vi "LickSpoutPrimer.vi"() -> ()   [LabVIEW 2019]
doc: "The myRIO Project template acquires acceleration data from the onboard accelerometer and displays the changes of acceleration values in a waveform chart."
uses:
  <vilib>/myRIO/Common/Instrument Driver Framework/myRIO v1.0/Encoder/typedefs/Encoder Signal Mode.ctl
  <vilib>/myRIO/Instrument Drivers/Onboard IO/Encoder/typedefs/Encoder Reference.ctl
  <vilib>/myRIO/Common/Instrument Driver Framework/Utilities/typedefs/myRIO Generic Hardware Reference.ctl
  <vilib>/myRIO/Common/Instrument Driver Framework/Utilities/typedefs/Hardware Version Enum.ctl
  <vilib>/myRIO/Common/Instrument Driver Framework/Utilities/typedefs/myRIO v1.0 Reference.ctl
  <vilib>/myRIO/Common/Instrument Driver Framework/Utilities/typedefs/Generic FPGA Reference.ctl
  <vilib>/myRIO/Common/Instrument Driver Framework/myRIO v1.0/Encoder/typedefs/Encoder Channels Enum.ctl
  <vilib>/myRIO/Common/Instrument Driver Framework/myRIO v1.0/Encoder/typedefs/Encoder Configuration v1.0.ctl
  <vilib>/userdefined/High Color/nirio_resource_hc.ctl
  <vilib>/myRIO/Instrument Drivers/Onboard IO/DIO/typedefs/DIO Reference.ctl
  <vilib>/myRIO/Common/Instrument Driver Framework/myRIO v1.0/DIO/typedefs/DIO Channels List.ctl
  <vilib>/myRIO/Common/Instrument Driver Framework/myRIO v1.0/DIO/typedefs/DIO Channels Enum.ctl
  <vilib>/myRIO/Common/Instrument Driver Framework/Utilities/vis/Is FPGA Ref Available.vi
  <vilib>/myRIO/Common/Instrument Driver Framework/myRIO v1.0/Encoder/vis/myRIO v1.1 Open Encoder.vi
  <vilib>/myRIO/Instrument Drivers/Onboard IO/Encoder/vis/Read.vi
  <vilib>/myRIO/Common/Instrument Driver Framework/myRIO v1.0/DIO/vis/myRIO v1.1 Open DIO.vi
  <vilib>/myRIO/Instrument Drivers/Onboard IO/DIO/vis/Read.vi
  <vilib>/myRIO/Instrument Drivers/Onboard IO/DIO/vis/Write.vi
  <vilib>/myRIO/Common/Instrument Driver Framework/Utilities/vis/Validate Channels.vi
  <vilib>/myRIO/Common/Instrument Driver Framework/myRIO v1.0/Encoder/vis/myRIO v1.0 Reserve Encoder.vi
  <vilib>/myRIO/Common/Instrument Driver Framework/myRIO v1.0/DIO/vis/myRIO v1.0 Reserve DIO.vi
  <vilib>/myRIO/Common/Instrument Driver Framework/myRIO v1.0/Encoder/vis/myRIO v1.0 Build MUX Configuration Encoder.vi
  <vilib>/myRIO/Common/Instrument Driver Framework/myRIO v1.0/Resource Manager/vis/myRIO v1.0 Reserve Channel List.vi
  <vilib>/myRIO/Common/Instrument Driver Framework/myRIO v1.0/DIO/vis/myRIO v1.0 Build MUX Configuration DIO.vi
  <vilib>/myRIO/Common/Instrument Driver Framework/myRIO v1.0/Resource Manager/vis/myRIO v1.0 Create Configuration List.vi
  <vilib>/myRIO/Common/Instrument Driver Framework/myRIO v1.0/Resource Manager/vis/myRIO v1.0 Reserve Channel.vi
  <vilib>/myRIO/Common/Instrument Driver Framework/myRIO v1.0/Resource Manager/vis/myRIO v1.0 Unreserve Channel.vi
  <vilib>/myRIO/Common/Instrument Driver Framework/myRIO v1.0/Resource Manager/vis/myRIO v1.0 Build Mutex Name.vi
  <vilib>/Utility/VariantDataType/GetNumericInfo.vi
  <vilib>/Utility/error.llb/Error Cluster From Error Code.vi
  <vilib>/myRIO/Common/Instrument Driver Framework/myRIO v1.0/myRIO v1.1 Open.vi
  <vilib>/myRIO/Common/Instrument Driver Framework/Utilities/vis/IO Manager.vi
  <vilib>/myRIO/Common/Instrument Driver Framework/Utilities/vis/Configuration Manager.vi
  <vilib>/myRIO/Common/Instrument Driver Framework/myRIO v1.0/Resource Manager/vis/myRIO v1.0 Configure IO.vi
  <vilib>/myRIO/Common/Instrument Driver Framework/myRIO v1.0/myRIO v1.0 Close.vi
  <vilib>/myRIO/Common/Instrument Driver Framework/myRIO v1.0/Encoder/vis/myRIO v1.0 Configure Encoder.vi
  <vilib>/myRIO/Common/Instrument Driver Framework/myRIO v1.0/Encoder/vis/myRIO v1.0 Read Encoder.vi
  <vilib>/myRIO/Common/Instrument Driver Framework/myRIO v1.0/DIO/vis/myRIO v1.0 Read DIO.vi
  <vilib>/myRIO/Common/Instrument Driver Framework/myRIO v1.0/DIO/vis/myRIO v1.0 Write DIO.vi
  <vilib>/myRIO/Express VI/Onboard IO/Encoder/Encoder Express VI.xnode
  <vilib>/myRIO/Instrument Drivers/Onboard IO/Encoder/vis/myRIO Encoder Open.xnode
  <vilib>/myRIO/Express VI/Onboard IO/DI/DI Express VI.xnode
  <vilib>/myRIO/Instrument Drivers/Onboard IO/DIO/vis/myRIO DIO Open.xnode
  <vilib>/myRIO/Express VI/Onboard IO/DO/DO Express VI.xnode
  <vilib>/myRIO/Instrument Drivers/Onboard IO/Encoder/Encoder.lvlib
  <vilib>/myRIO/Instrument Drivers/Onboard IO/DIO/DIO.lvlib
panel:
  in  "Stop Button":bool
  out "Time since last reward":dbl
  out "Time of last reward":dbl
  out "Rewards":u16
  out "Frame clock":i32
  out "Frames":u32
  out "Reward":bool=TRUE
  in  "Give reward":bool
  out "Licks":u32
  out "Lick":bool
  out "Output":dbl[][](array[numeric])
  out "Time":dbl
  out "Display":bool
  out "Overflow?":bool
  out "Counter Value":i32
  out "Velocity":dbl
  out "Velocity Plot":dbl[](graph)
  out "Velocity array":dbl[](array[numeric])
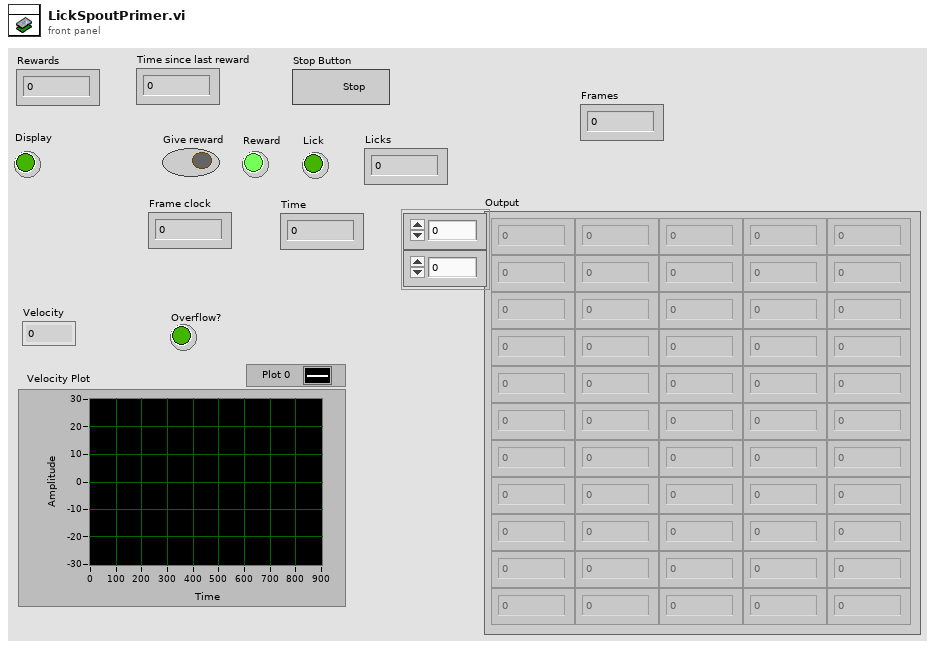
[diagram p1: front panel]
types:
  T1 = typedef "Encoder.lvlib/Encoder Reference.ctl" = cluster{"myRIO Reference":T2, "Encoder Channels Enum":T6}
  T2 = typedef "myRIO Generic Hardware Reference.ctl" = cluster{"myRIO Model":T3, "myRIO Hardware Reference":T4}
  T3 = typedef "Hardware Version Enum.ctl" = enum16{"Unknown", "myRIO-1900", "myRIO-1950", "roboRIO", "NI ELVIS RIO CM", "ELVIS III"}
  T4 = typedef "myRIO v1.0 Reference.ctl" = cluster{"Generic FPGA Reference":T5, "Allow multiple opens":bool}
  T5 = typedef "Generic FPGA Reference.ctl" = refnum<k20>
  T6 = typedef "Encoder Channels Enum.ctl" = enum16{"Not Connected", "C/ENC0", "C/ENC1", "A/ENC", "A/ENC0", "A/ENC1", "A/ENC2", "A/ENC3", "A/ENC4", "A/ENC5", "A/ENC6", "A/ENC7", "A/ENC8", "A/ENC9", "B/ENC", "B/ENC0", "B/ENC1", "B/ENC2", "B/ENC3", "B/ENC4", "B/ENC5", "B/ENC6", "B/ENC7", "B/ENC8", "B/ENC9", "DIO/ENC0", "DIO/ENC1", "DIO/ENC2", "DIO/ENC3", "DIO/ENC4"}
  T7 = typedef "Encoder Signal Mode.ctl" = enum16{"Quadrature phase signal", "Step and direction signal"}
  T8 = typedef "nirio_resource_hc.ctl" = tag
  T9 = typedef "DIO.lvlib/DIO Reference.ctl" = cluster{"myRIO Reference":T2, "DIO Channels List":T10}
  T10 = typedef "DIO Channels List.ctl" = T11[]
  T11 = typedef "DIO Channels Enum.ctl" = enum16{"Not Connected", "C/DIO0", "C/DIO1", "C/DIO2", "C/DIO3", "C/DIO4", "C/DIO5", "C/DIO6", "C/DIO7", "A/DIO0", "A/DIO1", "A/DIO2", "A/DIO3", "A/DIO4", "A/DIO5", "A/DIO6", "A/DIO7", "A/DIO8", "A/DIO9", "A/DIO10", "A/DIO11", "A/DIO12", "A/DIO13", "A/DIO14", "A/DIO15", "A/DIO16", "A/DIO17", "A/DIO18", "A/DIO19", "B/DIO0", "B/DIO1", "B/DIO2", "B/DIO3", "B/DIO4", "B/DIO5", "B/DIO6", "B/DIO7", "B/DIO8", "B/DIO9", "B/DIO10", "B/DIO11", "B/DIO12", "B/DIO13", "B/DIO14", "B/DIO15", "B/DIO16", "B/DIO17", "B/DIO18", "B/DIO19", "LED0", "LED1", "LED2", "LED3", "Button0", "DIO/DIO0", "DIO/DIO1", "DIO/DIO2", "DIO/DIO3", "DIO/DIO4", "DIO/DIO5", "DIO/DIO6", "DIO/DIO7", "DIO/DIO8", "DIO/DIO9", "SPI/CS0", "SPI/CS1", "SPI/CS2", "SPI/CS3", "LED RADIO (Green)", "LED RADIO (Red)", "LED COMM (Green)", "LED COMM (Red)", "LED MODE (Green)", "LED MODE (Red)"}
  T12 = typedef "NI_Matrix.lvlib/RealMatrix.ctl" = dbl[][]
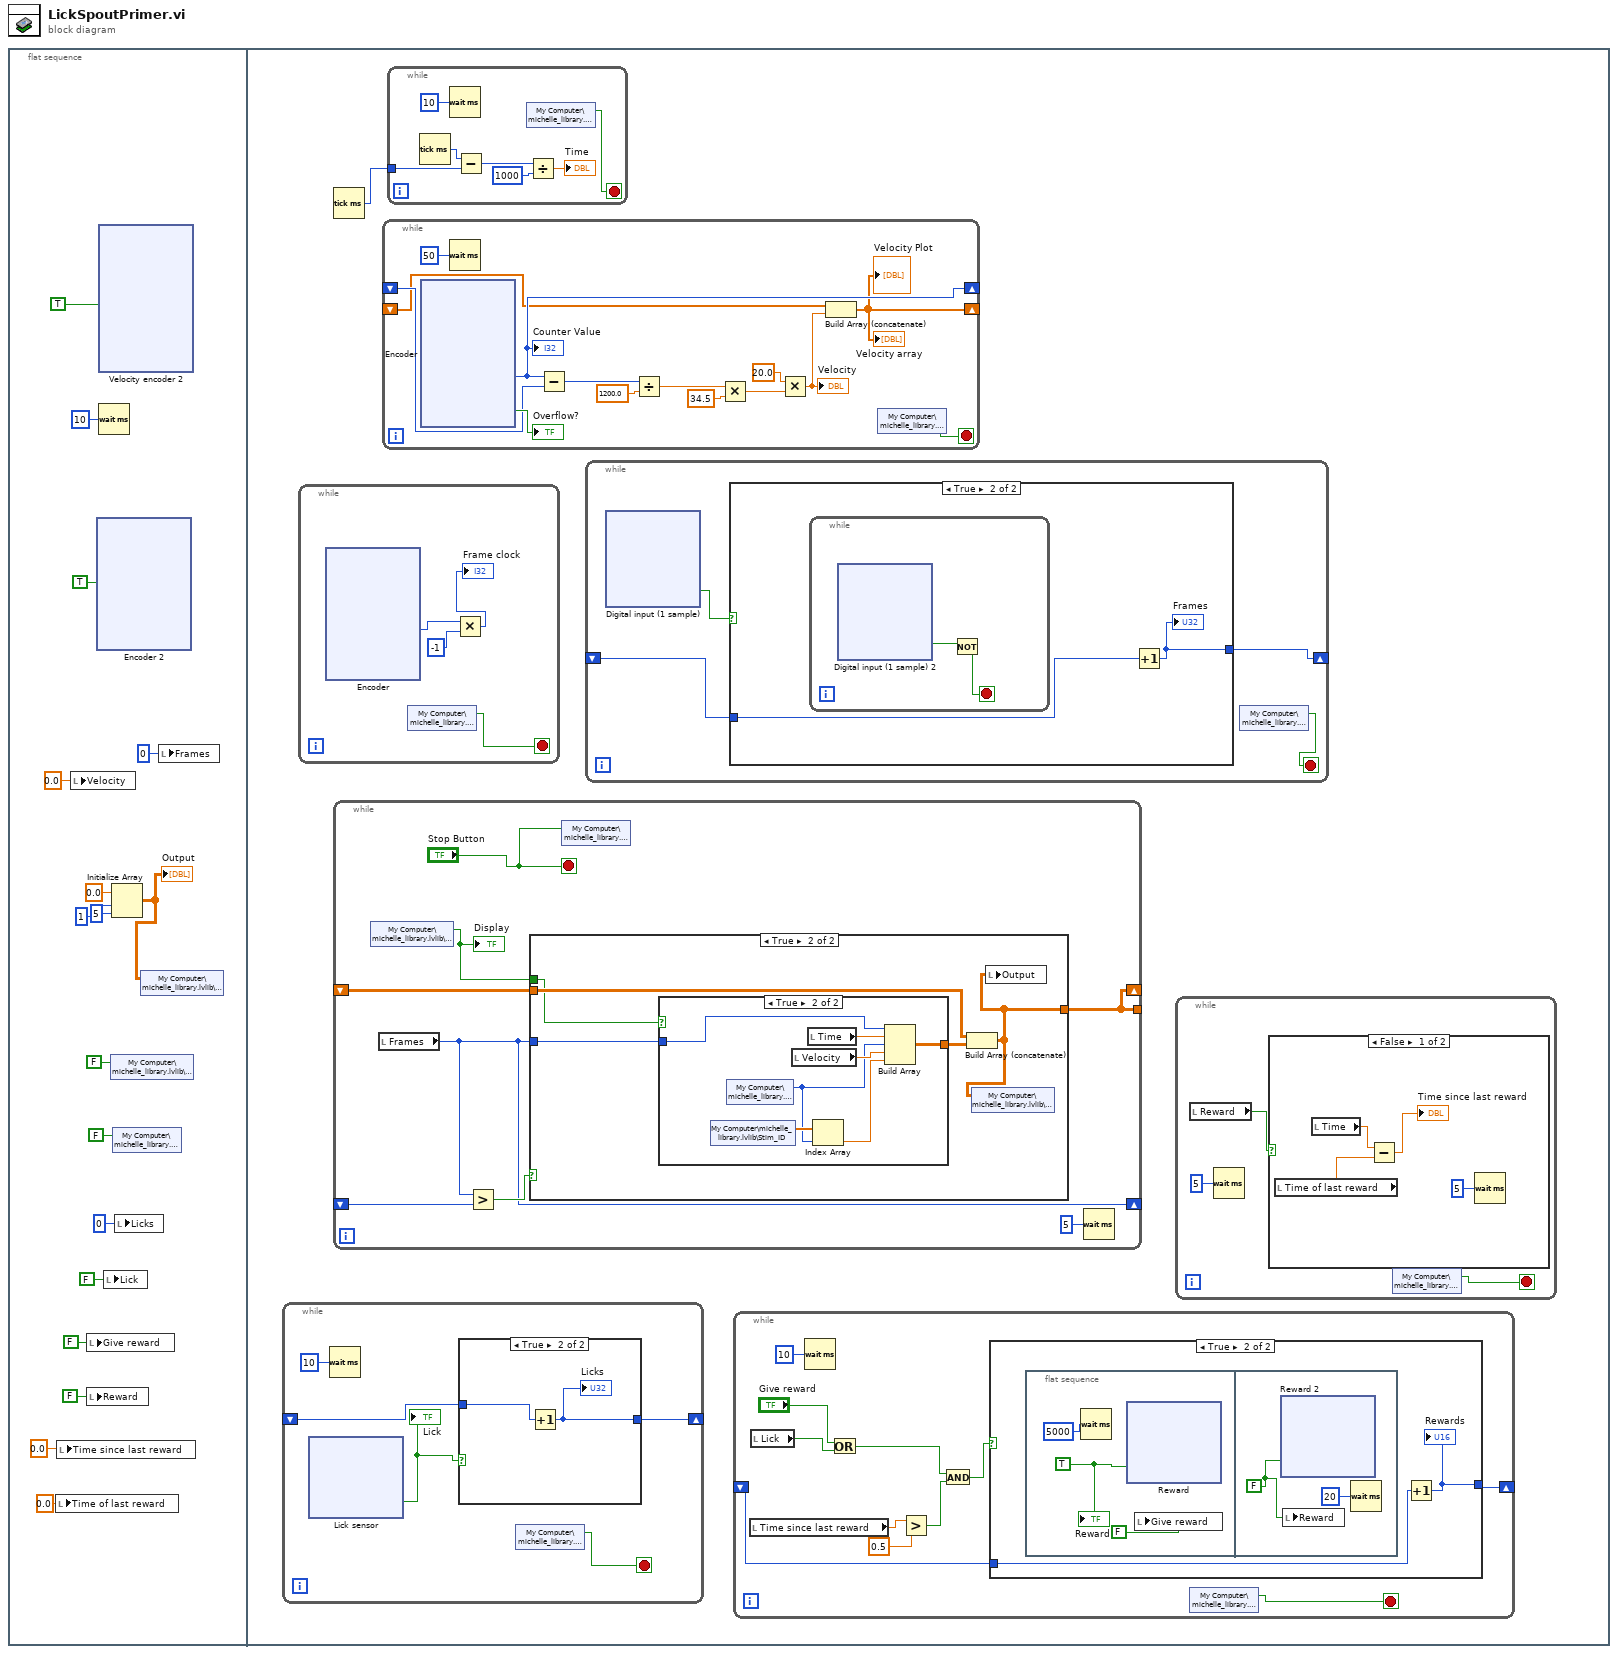
[diagram p0: block diagram]
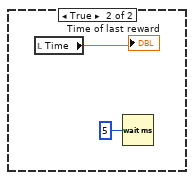
[diagram p2: hidden frame]
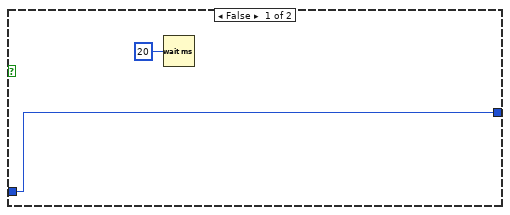
[diagram p4: hidden frame]
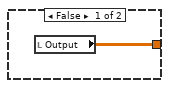
[diagram p6: hidden frame]
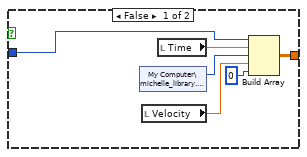
[diagram p7: hidden frame]
diagram:
  n1 = flat-sequence {
    frame #0 {
      n2 = local write "Time of last reward"(0.0 ("Time of last reward")) -> ()
      n3 = local write "Time since last reward"(0.0 ("Time since last reward")) -> ()
      n4 = local write "Velocity"(0.0 ("Velocity")) -> ()
      n5 = local write "Give reward"(FALSE ("Give reward")) -> ()
      n6 = local write "Reward"(FALSE ("Reward")) -> ()
      n7 = xnode "Encoder 2"("Reset Counter"=TRUE) -> ()  [unwired: 1 in, 4 out]
      n8 = xnode "Velocity encoder 2"("Reset Counter"=TRUE) -> ()  [unwired: 1 in, 4 out]
      n9 = Wait (ms)(milliseconds to wait=u32 10) -> ()  [unwired: 1 out]
      n10 = local write "Lick"(FALSE ("Lick")) -> ()
      n11 = shared-variable "My Computer\\michelle_library.lvlib\\Display"(FALSE ("Display")) -> ()  [unwired: 1 in, 1 out]
      n12 = Initialize Array(0.0 ("element"), 1 ("dimension size"), 5 ("dimension size")) -> (w11:dbl[][])
      "Output" <- w11
      n13 = shared-variable "My Computer\\michelle_library.lvlib\\Stop"(FALSE ("Stop")) -> ()  [unwired: 1 in, 1 out]
      n14 = local write "Licks"(u32 0 ("Licks")) -> ()
      n15 = shared-variable "My Computer\\michelle_library.lvlib\\Output"(w11) -> ()  [unwired: 1 in, 1 out]
      n16 = local write "Frames"(u32 0 ("Frames")) -> ()
    }
    frame #1 {
      n17 = while {
        shift-right: [w340] -> _
        shift-left: _ -> [w339]
        stop <- w343 stop-if-true
        n18 = xnode "Lick sensor"() -> ("C/DIO1 (DIO1)"=w341:bool)  [unwired: 1 in, 1 out]
        "Lick" <- w341
        n19 = Wait (ms)(milliseconds to wait=u32 10) -> ()  [unwired: 1 out]
        n20 = case shown="True" w341 {
          tunnel: [w344 w346] -> w340
          tunnel: w339 -> [w344 w345]
          frame False {
          }
          frame True {
            n21 = Increment(x=w345) -> (x+1=w346:u32)
            "Licks" <- w346
          }
        }
        n22 = shared-variable "My Computer\\michelle_library.lvlib\\Stop"() -> (w343:bool)  [unwired: 1 in, 1 out]
      }
      n23 = while {
        stop <- w120 stop-if-true
        n24 = xnode "Encoder"() -> ("Counter Value"=w123:i32)  [unwired: 2 in, 3 out]
        n25 = shared-variable "My Computer\\michelle_library.lvlib\\Stop"() -> (w120:bool)  [unwired: 1 in, 1 out]
        n26 = Multiply(x=w123, y=-1) -> (x*y=→"Frame clock":i32)
      }
      n27 = Tick Count (ms)() -> (millisecond timer value=w110:u32)
      n28 = while {
        shift-right: [w454] -> _
        shift-left: _ -> [w456]
        shift-right: [w451] -> _
        shift-left: _ -> [w453]
        tunnel: [w451] -> _
        stop <- "Stop Button" stop-if-true
        n29 = shared-variable "My Computer\\michelle_library.lvlib\\Display"() -> (w450:bool)  [unwired: 1 in, 1 out]
        "Display" <- w450
        n30 = local read "Frames"() -> (w454:u32)
        n31 = Greater?(x=w454, y=w456) -> (0:w455:bool)
        n32 = case shown="True" w455 {
          tunnel: w454 -> [_ w462]
          tunnel: w453 -> [_ w461]
          tunnel: [w457 w458] -> w451
          tunnel: w450 -> [_ w459]
          frame False {
            n33 = local read "Output"() -> (w457:dbl[][])
          }
          frame True {
            n34 = case shown="True" w459 {
              tunnel: w462 -> [w463 w475]
              tunnel: [w467 w474] -> w460
              frame False {
                n35 = shared-variable "My Computer\\michelle_library.lvlib\\Trial"() -> (w465:u32)  [unwired: 1 in, 1 out]
                n36 = local read "Velocity"() -> (w464:dbl)
                n37 = local read "Time"() -> (w466:dbl)
                n38 = Build Array(w463, w466, w465, w464, 0) -> (w467:T12)
              }
              frame True {
                n39 = shared-variable "My Computer\\michelle_library.lvlib\\Stim_ID"() -> (w471:dbl[])  [unwired: 1 in, 1 out]
                n40 = shared-variable "My Computer\\michelle_library.lvlib\\Trial"() -> (w470:u32)  [unwired: 1 in, 1 out]
                n41 = local read "Velocity"() -> (w472:dbl)
                n42 = local read "Time"() -> (w473:dbl)
                n43 = Index Array(array=w471, index=w470) -> (element=w469:dbl)
                n44 = Build Array(w475, w473, w470, w472, w469) -> (w474:T12)
              }
            }
            n45 = Build Array (concatenate)(w461, w460) -> (w458:T12)
            n46 = shared-variable "My Computer\\michelle_library.lvlib\\Output"(w458) -> ()  [unwired: 1 in, 1 out]
            n47 = local write "Output"(w458) -> ()
          }
        }
        n48 = shared-variable "My Computer\\michelle_library.lvlib\\Stop"("Stop Button") -> ()  [unwired: 1 in, 1 out]
        n49 = Wait (ms)(milliseconds to wait=u32 5) -> ()  [unwired: 1 out]
      }
      n50 = while {
        shift-right: [w392] -> _
        shift-left: _ -> [w393]
        shift-right: [w384] -> _
        shift-left: _ -> [w383]
        stop <- w382 stop-if-true
        n51 = xnode "Encoder"() -> ("Counter Value"=w392:i32, "Overflow?"=→"Overflow?":bool)  [unwired: 2 in, 2 out]
        "Counter Value" <- w392
        n52 = Wait (ms)(milliseconds to wait=u32 50) -> ()  [unwired: 1 out]
        n53 = Subtract(x=w392, y=w393) -> (x-y=w385:i32)
        n54 = Divide(x=w385, y=1200.0 ("600")) -> (x/y=w390:dbl)
        n55 = Multiply(x=w390, y=34.5) -> (x*y=w388:dbl)
        n56 = Multiply(x=20.0, y=w388) -> (x*y=w386:dbl)
        "Velocity" <- w386
        n57 = Build Array (concatenate)(w383, w386) -> (w384:dbl[])
        "Velocity Plot" <- w384
        "Velocity array" <- w384
        n58 = shared-variable "My Computer\\michelle_library.lvlib\\Stop"() -> (w382:bool)  [unwired: 1 in, 1 out]
      }
      n59 = while {
        tunnel: w110 -> [w447]
        stop <- w442 stop-if-true
        n60 = Tick Count (ms)() -> (millisecond timer value=w448:u32)
        n61 = Wait (ms)(milliseconds to wait=u32 10) -> ()  [unwired: 1 out]
        n62 = Subtract(x=w448, y=w447) -> (x-y=w445:u32)
        n63 = shared-variable "My Computer\\michelle_library.lvlib\\Stop"() -> (w442:bool)  [unwired: 1 in, 1 out]
        n64 = Divide(x=w445, y=u32 1000) -> (x/y=→"Time":dbl)
      }
      n65 = while {
        shift-right: [w173] -> _
        shift-left: _ -> [w172]
        stop <- w171 stop-if-true
        n66 = xnode "Digital input (1 sample)"() -> ("A/DIO13 (Pin 26)"=w170:bool)  [unwired: 1 in, 1 out]
        n67 = case shown="True" w170 {
          tunnel: [w209 w211] -> w173
          tunnel: w172 -> [w209 w210]
          frame False {
          }
          frame True {
            n68 = while {
              stop <- w213 stop-if-true
              n69 = xnode "Digital input (1 sample) 2"() -> ("A/DIO13 (Pin 26)"=w212:bool)  [unwired: 1 in, 1 out]
              n70 = Not(x=w212) -> (.not. x?=w213:bool)
            }
            n71 = Increment(x=w210) -> (x+1=w211:u32)
            "Frames" <- w211
          }
        }
        n72 = shared-variable "My Computer\\michelle_library.lvlib\\Stop"() -> (w171:bool)  [unwired: 1 in, 1 out]
      }
      n73 = while {
        shift-right: [w258] -> _
        shift-left: _ -> [w257]
        stop <- w259 stop-if-true
        n74 = local read "Time since last reward"() -> (w253:dbl)
        n75 = local read "Lick"() -> (w255:bool)
        n76 = Wait (ms)(milliseconds to wait=u32 10) -> ()  [unwired: 1 out]
        n77 = Or(x="Give reward", y=w255) -> (x .or. y?=w250:bool)
        n78 = Greater?(x=w253, y=0.5) -> (0:w251:bool)
        n79 = And(x=w250, y=w251) -> (x .and. y?=w249:bool)
        n80 = case shown="True" w249 {
          tunnel: [w261 w263] -> w258
          tunnel: w257 -> [w261 w262]
          frame False {
            n81 = Wait (ms)(milliseconds to wait=u32 20) -> ()  [unwired: 1 out]
          }
          frame True {
            n82 = flat-sequence {
              frame #0 {
                w266 = TRUE ("C/DIO0 (DIO0)")
                n83 = Wait (ms)(milliseconds to wait=u32 5000) -> ()  [unwired: 1 out]
                n84 = xnode "Reward"("C/DIO0 (DIO0)"=w266) -> ()  [unwired: 1 in, 1 out]
                n85 = local write "Give reward"(FALSE ("Give reward")) -> ()
                "Reward" <- w266
              }
              frame #1 {
                w303 = FALSE ("C/DIO0 (DIO0)")
                n86 = xnode "Reward 2"("C/DIO0 (DIO0)"=w303) -> ()  [unwired: 1 in, 1 out]
                n87 = local write "Reward"(w303) -> ()
                n88 = Wait (ms)(milliseconds to wait=u32 20) -> ()  [unwired: 1 out]
              }
            }
            n89 = Increment(x=w262) -> (x+1=w263:u16)
            "Rewards" <- w263
          }
        }
        n90 = shared-variable "My Computer\\michelle_library.lvlib\\Stop"() -> (w259:bool)  [unwired: 1 in, 1 out]
      }
      n91 = while {
        stop <- w111 stop-if-true
        n92 = local read "Reward"() -> (w113:bool)
        n93 = Wait (ms)(milliseconds to wait=u32 5) -> ()  [unwired: 1 out]
        n94 = case shown="False" w113 {
          frame False {
            n95 = local read "Time of last reward"() -> (w115:dbl)
            n96 = local read "Time"() -> (w116:dbl)
            n97 = Subtract(x=w116, y=w115) -> (x-y=→"Time since last reward":dbl)
            n98 = Wait (ms)(milliseconds to wait=u32 5) -> ()  [unwired: 1 out]
          }
          frame True {
            n99 = local read "Time"() -> (→"Time of last reward":dbl)
            n100 = Wait (ms)(milliseconds to wait=u32 5) -> ()  [unwired: 1 out]
          }
        }
        n101 = shared-variable "My Computer\\michelle_library.lvlib\\Stop"() -> (w111:bool)  [unwired: 1 in, 1 out]
      }
    }
  }
